vi "ITX to HDF5.vi"(8 "error in (no error)":errorcluster, 10 "file (use dialog)":path=path "P:/sample/GaAs/GaAs quantum dots/2008/PL Map/A1 735/060731ASBA_A1_6.0.itx", 11 "LVtoITX in":refnum<class "LVtoITX.lvclass">) -> (0 "error out":errorcluster, 3 "LVtoITX out":refnum<class "LVtoITX.lvclass">)   [LabVIEW 2016, in "LVtoITX.lvclass"]
uses:
  LVtoITX.lvclass
  LVtoITX.lvclass/LVtoITX.ctl
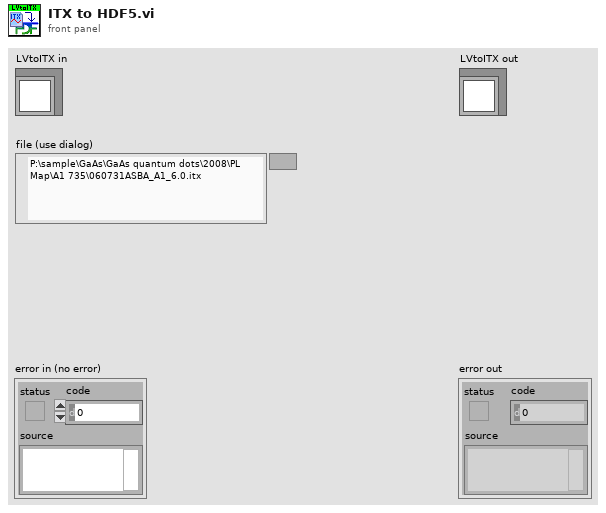
[diagram p1: front panel]
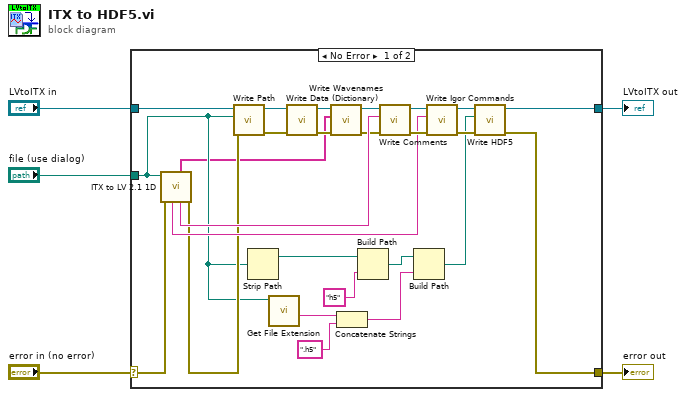
[diagram p0: block diagram]
diagram:
  n1 = case shown="No Error" "error in (no error)" {
    selector: "error in (no error)" -> [w31 w33]
    tunnel: [w16 w33] -> w4
    tunnel: [w15 w32] -> w2
    tunnel: "LVtoITX in" -> [w29 w32]
    tunnel: "file (use dialog)" -> [w12 _]
    frame No Error {
      n2 = call "ITX to LV 2.1 1D.vi"("error in"=w31, "file (use dialog)"=w12) -> ("error out"=w17:errorcluster, "Notes"=w30:string, "base wavenames"=w6:string[], "Commands"=w20:string)  [unwired: 4 in, 2 out]
      n3 = call "Write Path.vi"("error in (no error)"=w17, "Path"=w12, "LVtoITX in"=w29) -> ("error out"=w27:errorcluster, "LVtoITX out"=w28:refnum<class "LVtoITX.lvclass">)  [unwired: 7 in]
      n4 = Strip Path(path=w12) -> (stripped path=w7:path)  [unwired: 1 out]
      n5 = call <vilib>:"Get File Extension.vi"("file"=w12) -> ("filename without extension"=w14:string)  [unwired: 6 in, 4 out]
      n6 = call "Write Data (Dictionary).vi"("error in (no error)"=w27, "LVtoITX in"=w28) -> ("error out"=w25:errorcluster, "LVtoITX out"=w26:refnum<class "LVtoITX.lvclass">)  [unwired: 8 in]
      n7 = call "Write Wavenames.vi"("error in (no error)"=w25, "Wavenames"=w6, "LVtoITX in"=w26) -> ("error out"=w23:errorcluster, "LVtoITX out"=w24:refnum<class "LVtoITX.lvclass">)  [unwired: 7 in]
      n8 = Concatenate Strings(w14, ".h5" ("string")) -> (w13:string)
      n9 = Build Path(base path=w7, name or relative path="h5" ("string")) -> (appended path=w8:path)
      n10 = call "Write Comments.vi"("error in (no error)"=w23, "Comments"=w30, "LVtoITX in"=w24) -> ("error out"=w21:errorcluster, "LVtoITX out"=w22:refnum<class "LVtoITX.lvclass">)  [unwired: 7 in]
      n11 = Build Path(base path=w8, name or relative path=w13) -> (appended path=w11:path)
      n12 = call "Write Igor Commands.vi"("error in (no error)"=w21, "Igor Commands"=w20, "LVtoITX in"=w22) -> ("error out"=w18:errorcluster, "LVtoITX out"=w19:refnum<class "LVtoITX.lvclass">)  [unwired: 7 in]
      n13 = call "Write HDF5.vi"("error in (no error)"=w18, "path"=w11, "LVtoITX in"=w19) -> ("error out"=w16:errorcluster, "LVtoITX out"=w15:refnum<class "LVtoITX.lvclass">)  [unwired: 7 in]
    }
    frame Error {
    }
  }
  "error out" <- w4
  "LVtoITX out" <- w2
